vi "SPC_get_error_string.vi"(6 "ErrorID":i16, 7 "VI-name if Inline":string, 8 "Error In":errorcluster, 11 "DLL Path":path) -> (0 "Error Out":errorcluster, 2 "ErrorID":i16, 3 "DLL Path":path)   [LabVIEW 2023]
doc: "The procedure copies the string which contains the explanation of the SPC DLL error provided by 'error_id'to the LV ErrorCluster's source field.\nFor debugging aid, this VI adds the name of the calling VI (usually the LV-SPCM DLL wrapper) to the error description in the source field. \nWire manually the name of the wrapper to 'VI-name if Inline' when the wrapper's name can't be found on the Call Chain list. \n\ninfo@becker-hickl.com"
panel:
  out "Error String":string
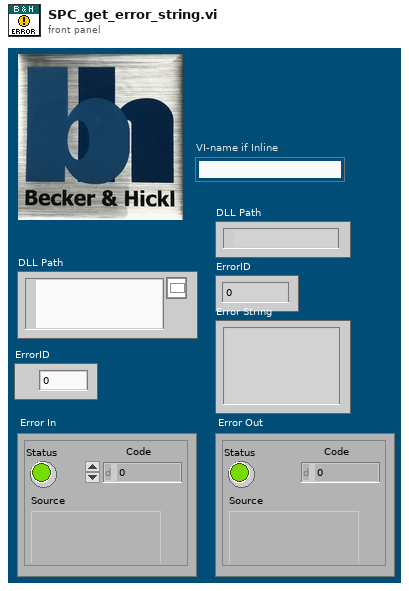
[diagram p1: front panel]
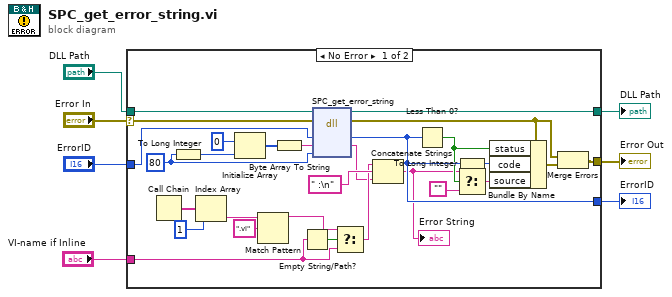
[diagram p0: block diagram]
diagram:
  n1 = case shown="No Error" "Error In" {
    selector: "Error In" -> [w35 w38]
    tunnel: [w11 w38] -> w6
    tunnel: [w34 w37] -> w5
    tunnel: "DLL Path" -> [w33 w37]
    tunnel: "ErrorID" -> [w32 w36]
    tunnel: [w24 w36] -> w2
    tunnel: "VI-name if Inline" -> [w12 _]
    frame No Error {
      w29 = i16 80 ("MaxLength")
      n2 = Call Chain() -> (call chain=w17:string[])
      n3 = To Long Integer(number=w29) -> (32bit integer=w28:i32)
      n4 = Index Array(array=w17, index=1) -> (element=w15:string)
      n5 = Initialize Array(u8 0, w28) -> (w26:u8[])
      n6 = Match Pattern(string=w15, regular expression=".vi") -> (before substring=w13:string)  [unwired: 1 in, 3 out]
      n7 = Byte Array To String(unsigned byte array=w26) -> (string=w25:string)
      n8 = Empty String/Path?(string/path=w12) -> (empty?=w14:bool)
      n9 = dll-call lib="C:/Program Files (x86)/BH/SPCM/DLL/spcm64.dll" fn="SPC_get_error_string"(path in=w33, error in=w35, "ErrorID"=w32, "ErrorString"=w25, "MaxLength"=w29) -> (path out=w34:path, error out=w10:errorcluster, "ErrorID"=w24:i16, "ErrorString"=w8:string)  [unwired: 3 in]
      n10 = Select(t=w13, s=w14, f=w12) -> (s? t:f=w9:string)
      n11 = Concatenate Strings(w9, " :\n" ("string"), w8) -> (w19:string)
      "Error String" <- w19
      n12 = Less Than 0?(x=w24) -> (x < 0?=w20:bool)
      n13 = To Long Integer(number=w24) -> (32bit integer=w30:i32)
      n14 = Select(t=w19, s=w20, f="") -> (s? t:f=w21:string)
      n15 = Bundle By Name(cluster=w10, "status"=w20, "code"=w30, "source"=w21) -> (w31:errorcluster)
      n16 = Merge Errors(w10, w31) -> (w11:errorcluster)
    }
    frame Error {
    }
  }
  "Error Out" <- w6
  "DLL Path" <- w5
  "ErrorID" <- w2
